vi "format set pattern.vi"(8 "error in (no error)":errorcluster, 10 "pattern":T1 items=["LXW_PATTERN_NONE", "LXW_PATTERN_SOLID", "LXW_PATTERN_MEDIUM_GRAY", "LXW_PATTERN_DARK_GRAY", "LXW_PATTERN_LIGHT_GRAY"], 11 "format":u32) -> (0 "error out":errorcluster)   [LabVIEW 2015, in "xlsxwriter.lvlib"]
doc: "void format_set_pattern(lxw_format format, uint8_t pattern);"
uses:
  xlsxwriter.lvlib
  Controls/lxw_pattern_type.ctl
  xlsxwriter.dll
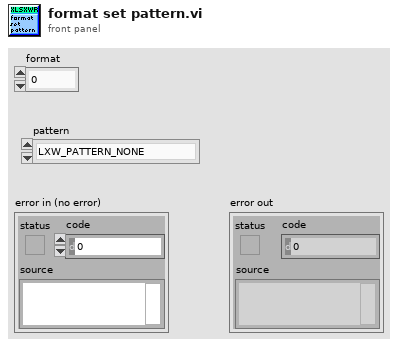
[diagram p1: front panel]
types:
  T1 = typedef "lxw_pattern_type.ctl" = u8
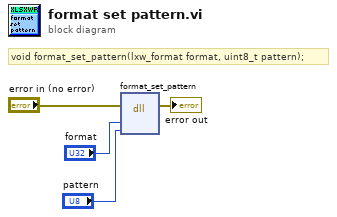
[diagram p0: block diagram]
diagram:
  # "void format_set_pattern(lxw_format format, uint8_t pattern);"
  n1 = dll-call lib="C:/Users/WDAGUtilityAccount/Desktop/Labview_Example-win32/xlsxwriter.*" fn="format_set_pattern"(error in="error in (no error)", "format"="format", "pattern"="pattern") -> (error out=→"error out":errorcluster)  [unwired: 5 in, 1 out]
